vi "Tools Dialog.vi"(7 "Settings":T1, 8 "Error In":errorcluster, 10 "Context":refnum<k7>, 11 "Tools In":refnum<class "Tools.lvclass">[](array[class])) -> (0 "Error Out":errorcluster, 1 "Canceled?":bool, 2 "ID":string, 3 "Tools Out":refnum<class "Tools.lvclass">[](array[class]))   [LabVIEW 2021, in "Seq Edit Quick Drop.lvlib"]
uses:
  Seq Edit Quick Drop.lvlib
  Dependencies/Tool Menu Utility.lvlibp/Tools/Tools.lvclass
  Control Keys.ctl
  Get Modifier.vi
  <vilib>/Utility/error.llb/Trim Whitespace.vi
  <vilib>/addons/TestStand/_TSUtility.llb/TestStand - End Modal Dialog (Sequence Context).vi
  <vilib>/addons/TestStand/_TSUtility.llb/TestStand - Start Modal Dialog (Sequence Context).vi
panel:
  in  "Parameters":string
  in  "Tools":string(tree)
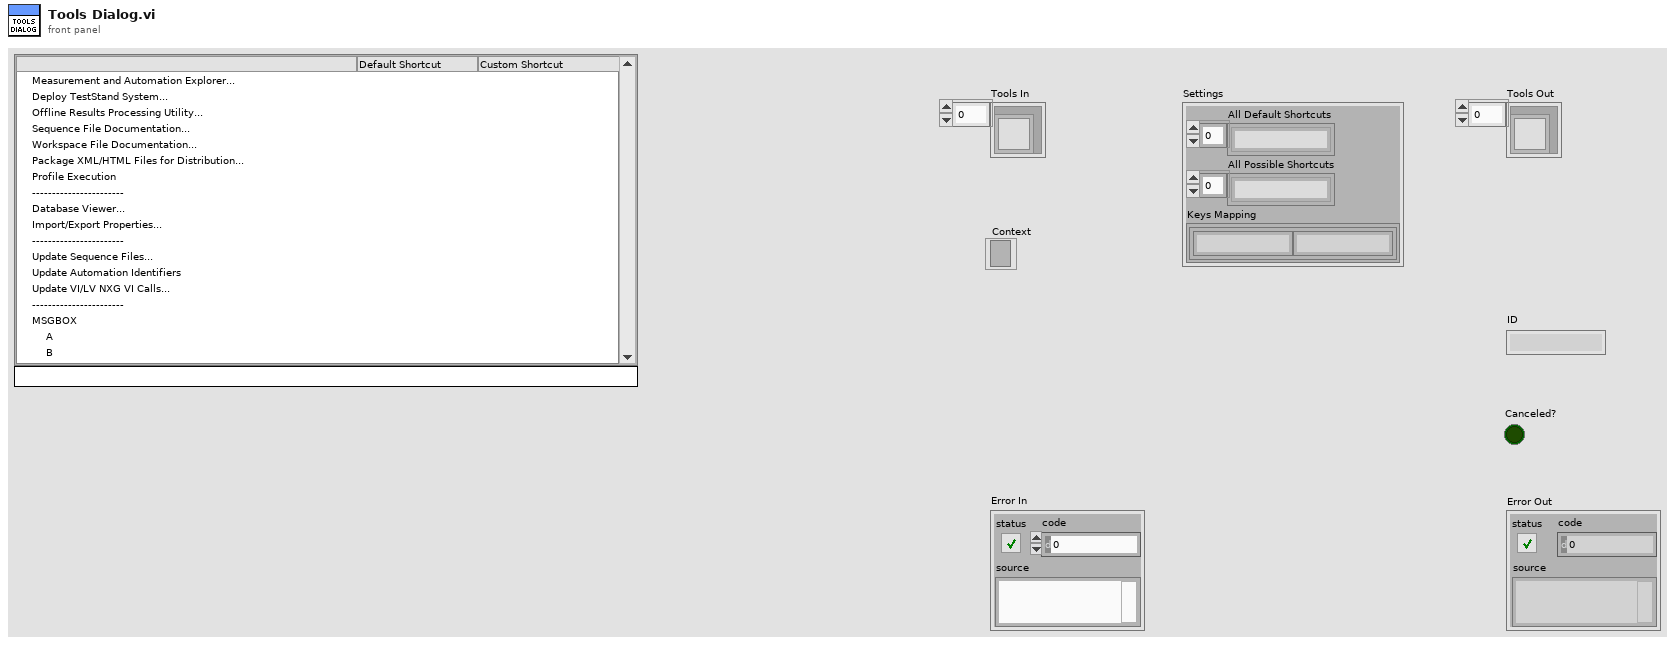
[diagram p1: front panel]
types:
  T1 = cluster{"All Default Shortcuts":string[], "All Possible Shortcuts":string[], "Keys Mapping":map{string, string}}
  T2 = typedef "Seq Edit Quick Drop.lvlib/Control Keys.ctl" = enum16{"Other", "Enter", "Escape", "Tab", "Up", "Down"}
  T3 = typedef "TestStand - Status Monitor.ctl" = cluster{"Sequence Context":refnum<k7>, "Execution":refnum<k7>, "Termination Monitor":refnum<k7>}
  T4 = cluster{"Shift":bool, "Ctrl":bool, "Alt":bool, "Cmd":bool, "Opt":bool}
  T5 = typedef "eventvkey.ctl" = enum16{"ASCII", "Enter", "Return", "Shift", "Ctrl", "Alt", "Cmd", "Opt", "Caps", "NumLock", "Clear", "Break", "Up", "Down", "Left", "Right", "Insert", "Delete", "Home", "End", "PageUp", "PageDown", "Escape", "Help", "Pause", "ScrollLock", "F1", "F2", "F3", "F4", "F5", "F6", "F7", "F8", "F9", "F10", "F11", "F12", "F13", "F14", "F15", "F16", "F17", "F18", "F19", "F20", "F21", "F22", "F23", "F24", "Play", "VolumeUp", "VolumeDown", "Mute", "Two Byte Char"}
  T6 = typedef "Seq Edit Quick Drop.lvlib/Modifiers.ctl" = enum16{"SHIFT", "CTRL", "ALT"}
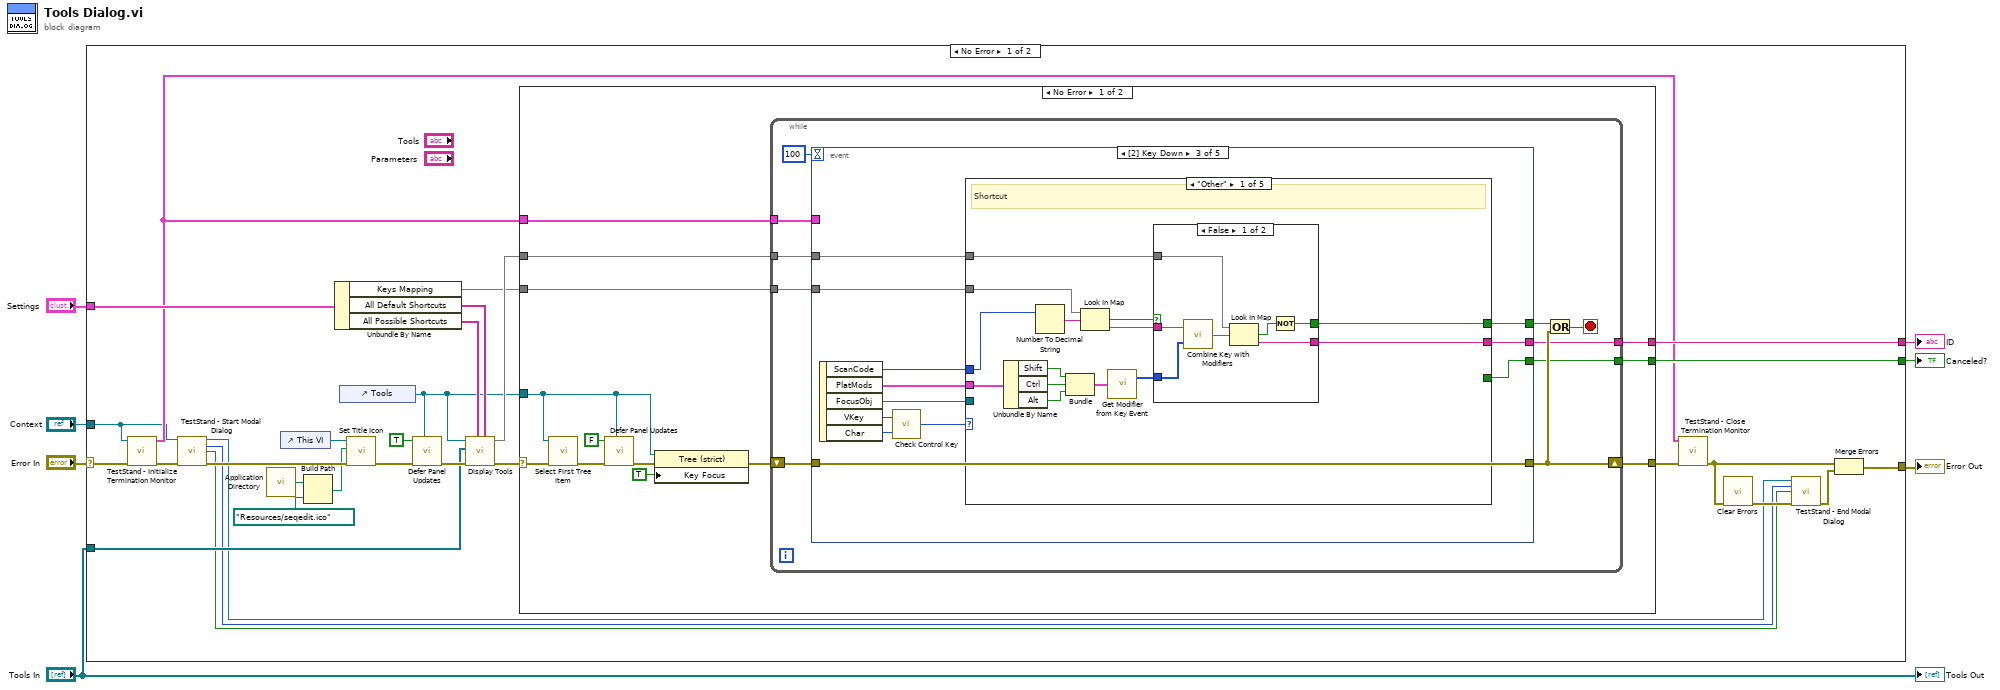
[diagram p0: block diagram]
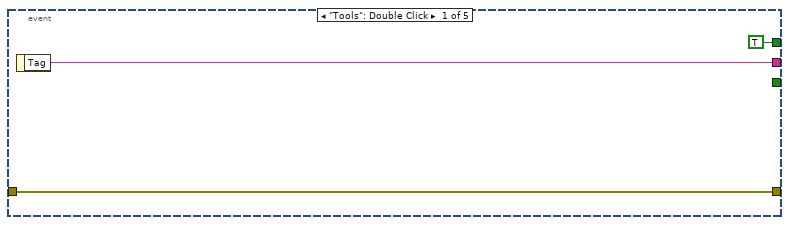
[diagram p2: hidden frame]
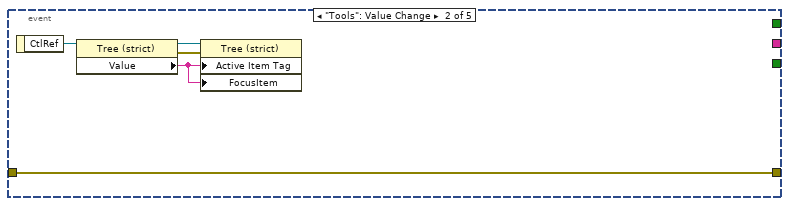
[diagram p3: hidden frame]
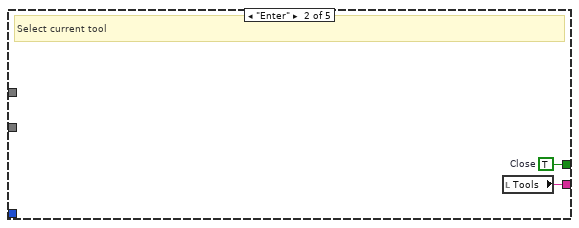
[diagram p5: hidden frame]
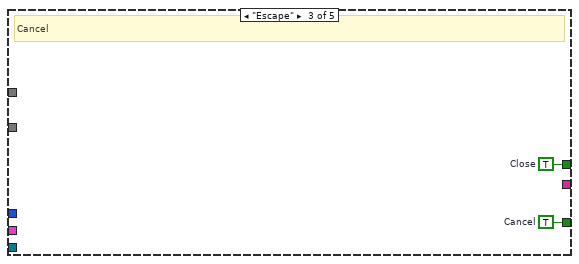
[diagram p6: hidden frame]
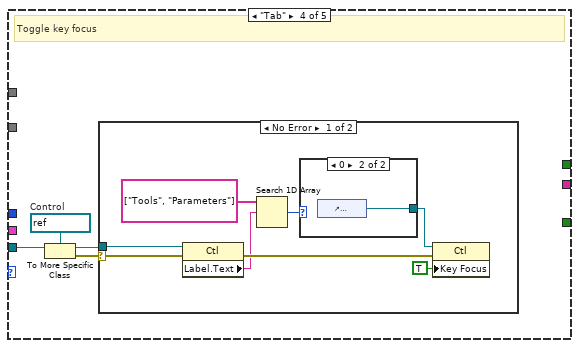
[diagram p7: hidden frame]
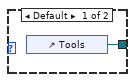
[diagram p8: hidden frame]
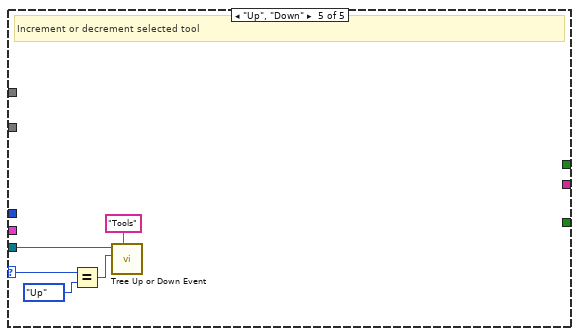
[diagram p10: hidden frame]
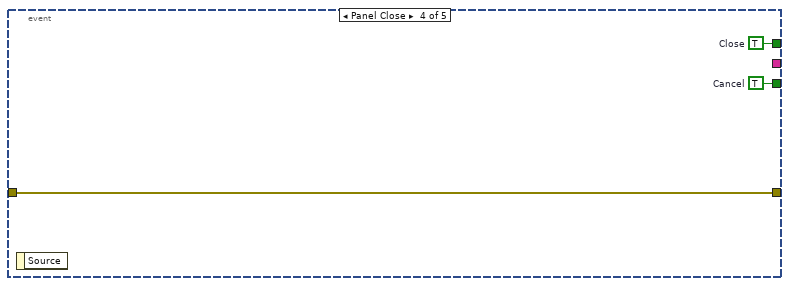
[diagram p11: hidden frame]
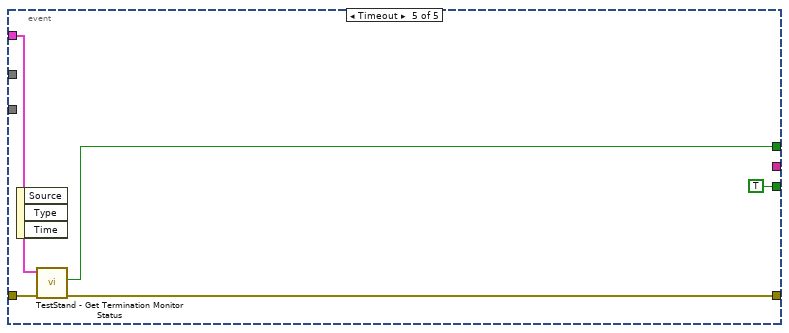
[diagram p12: hidden frame]
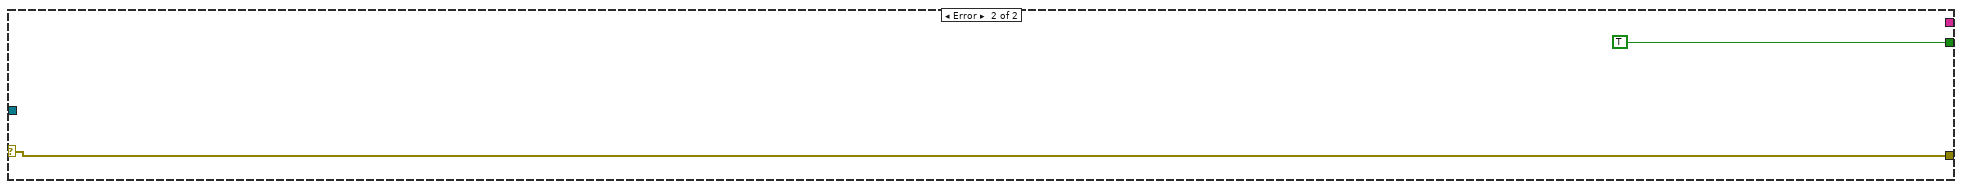
[diagram p14: hidden frame]
diagram:
  n1 = case shown="No Error" "Error In" {
    selector: "Error In" -> [w8 w135]
    tunnel: [w32 _] -> w7
    tunnel: "Tools In" -> [w31 _]
    tunnel: "Settings" -> [w30 _]
    tunnel: [w26 TRUE ("Cancel")] -> w4
    tunnel: [w24 w135] -> w3
    tunnel: "Context" -> [w14 _]
    frame No Error {
      n2 = call <vilib>:"TestStand - Initialize Termination Monitor.vi"("error in (no error)"=w8, "Sequence Context In"=w14) -> ("error out"=w21:errorcluster, "Status Monitor Out"=w19:T3)  [unwired: 8 in]
      n3 = call-poly <vilib>:"TestStand - Start Modal Dialog.vi"("Sequence Context In"=w14, "error in (no error)"=w21) -> ("Sequence Context Out"=w18:refnum<k7>, "Modal ID"=w23:i32, "VI Originally Open"=w22:bool, "error out"=w37:errorcluster)  [unwired: 9 in, 1 out]
      n4 = call <vilib>:"Application Directory.vi"() -> ("Application Directory"=w12:path)
      n5 = control-ref of="This VI"() -> (w13:refnum<vi>)
      n6 = Build Path(base path=w12, name or relative path=path "Resources/seqedit.ico") -> (appended path=w10:path)
      n7 = Unbundle By Name(w30) -> ("Keys Mapping"=w27:map{string, string}, "All Default Shortcuts"=w28:string[], "All Possible Shortcuts"=w29:string[])
      n8 = control-ref of="Tools"() -> (w15:refnum<vi>)
      n9 = call "Set Title Icon.vi"("Error In"=w37, "Icon Path"=w10, "VI Reference"=w13) -> ("Error Out"=w9:errorcluster)  [unwired: 8 in]
      n10 = call "Defer Panel Updates.vi"("Control"=w15, "Error In"=w9, "Defer Panel Updates"=TRUE) -> ("Error Out"=w34:errorcluster)  [unwired: 8 in]
      n11 = call "Display Tools.vi"("All Default Shortcuts"=w28, "All Possible Shortcuts"=w29, "Error In"=w34, "Tools"=w31, "Tools Tree Control"=w15) -> ("Error Out"=w35:errorcluster, "Shortcuts"=w33:map{string, string})  [unwired: 5 in]
      n12 = case shown="No Error" w35 {
        selector: w35 -> [w47 w133]
        tunnel: w33 -> [w49 _]
        tunnel: w15 -> [w41 _]
        tunnel: [w46 _] -> w32
        tunnel: w27 -> [w48 _]
        tunnel: [w45 _] -> w26
        tunnel: w19 -> [w39 _]
        tunnel: [w38 w133] -> w20
        frame No Error {
          n13 = call "Select First Tree Item.vi"("error in (no error)"=w47, "TreeControl in"=w41) -> ("error out"=w50:errorcluster)  [unwired: 8 in, 1 out]
          n14 = call "Defer Panel Updates.vi"("Control"=w41, "Error In"=w50, "Defer Panel Updates"=FALSE) -> ("Error Out"=w44:errorcluster)  [unwired: 8 in]
          n15 = property class="Tree (strict)"(reference=w41, error in=w44, "Key Focus"=TRUE) -> (error out=w42:errorcluster)  [unwired: 1 out]
          n16 = while {
            tunnel: [w59] -> w45
            tunnel: [w58] -> w46
            tunnel: w48 -> [w57]
            tunnel: w49 -> [w56]
            tunnel: w39 -> [w55]
            shift-right: [w60] -> w38
            shift-left: w42 -> [w53]
            stop <- w51 stop-if-true
            n17 = event shown="[2] Key Down" {
              selector: _ -> [_ _ _ _ _]
              dyn-events: _ -> [_ _ _ _ _]
              timeout: 100 -> [_ _ _ _ _]
              tunnel: [_ _ w75 w127 TRUE ("Cancel")] -> w59
              tunnel: [w63 _ w76 _ _] -> w58
              tunnel: w57 -> [_ _ w79 _ _]
              tunnel: [TRUE ("Close") _ w74 w126 w132] -> w52
              tunnel: w56 -> [_ _ w73 _ _]
              tunnel: w55 -> [_ _ _ _ w130]
              tunnel: w53 -> [w61 w64 w69 w125 w129]
              tunnel: [w61 w64 w69 w125 w128] -> w60
              event "Tools": Double Click {
                n18 = event-data() -> ("Tag"=w63:string)  [unwired: 1 in]
              }
              event "Tools": Value Change {
                n19 = event-data() -> ("CtlRef"=w68:refnum<vi>)  [unwired: 1 in]
                n20 = property class="Tree (strict)"(reference=w68) -> (reference out=w67:refnum<vi>, error out=w66:errorcluster, "Value"=w65:string)  [unwired: 1 in]
                n21 = property class="Tree (strict)"(reference=w67, error in=w66, "Active Item Tag"=w65, "FocusItem"=w65) -> ()  [unwired: 2 out]
              }
              event Key Down {
                n22 = event-data() -> ("ScanCode"=w80:i16, "PlatMods"=w78:T4, "FocusObj"=w70:refnum<vi>, "VKey"=w71:T5, "Char"=w72:i16)  [unwired: 1 in]
                n23 = call "Check Control Key.vi"("Char"=w72, "VKey"=w71) -> ("Control Key"=w77:T2)
                n24 = case shown="\"Other\"" w77 {
                  selector: w77 -> [_ _ _ _ w122]
                  tunnel: w80 -> [w94 _ _ _ _]
                  tunnel: w79 -> [w92 _ _ _ _]
                  tunnel: w78 -> [w88 _ _ _ _]
                  tunnel: [w82 w103 _ _ _] -> w76
                  tunnel: [_ _ w105 _ _] -> w75
                  tunnel: [w81 w102 w104 _ _] -> w74
                  tunnel: w70 -> [_ _ _ w109 w124]
                  tunnel: w73 -> [w83 _ _ _ _]
                  frame "Other" {
                    # "Shortcut"
                    n25 = Unbundle By Name(w88) -> ("Shift"=w87:bool, "Ctrl"=w86:bool, "Alt"=w85:bool)
                    n26 = Number To Decimal String(number=w94) -> (decimal integer string=w93:string)  [unwired: 1 in]
                    n27 = Bundle("Shift"=w87, "Ctrl"=w86, "Alt"=w85) -> (w84:cluster{"Shift":bool, "Ctrl":bool, "Alt":bool})  [unwired: 1 in]
                    n28 = Look In Map(map=w92, key=w93) -> (key not found?=w91:bool, value=w89:string)  [unwired: 1 in]
                    n29 = call "Get Modifier from Key Event.vi"("Modifiers"=w84) -> ("Modifiers"=w90:T6[])  [unwired: 1 out]
                    n30 = case shown="False" w91 {
                      tunnel: w90 -> [w101 _]
                      tunnel: w89 -> [w100 _]
                      tunnel: w83 -> [w98 _]
                      tunnel: [w97 _] -> w82
                      tunnel: [w95 _] -> w81
                      frame False {
                        n31 = call "Combine Key with Modifiers.vi"("Modifiers"=w101, "Key"=w100) -> ("Combined"=w99:string)
                        n32 = Look In Map(map=w98, key=w99) -> (key not found?=w96:bool, value=w97:string)  [unwired: 1 in]
                        n33 = Not(x=w96) -> (.not. x?=w95:bool)
                      }
                      frame True {
                      }
                    }
                  }
                  frame "Enter" {
                    w102 = TRUE  # Close
                    # "Select current tool"
                    n34 = local read "Tools"() -> (w103:string)
                  }
                  frame "Escape" {
                    w104 = TRUE  # Close
                    w105 = TRUE  # Cancel
                    # "Cancel"
                  }
                  frame "Tab" {
                    w108 = refnum<vi> refnum  # Control
                    # "Toggle key focus"
                    n35 = To More Specific Class(target class=w108, reference=w109) -> (specific class reference=w106:refnum<vi>, error out=w107:errorcluster)  [unwired: 1 in]
                    n36 = case shown="No Error" w107 {
                      selector: w107 -> [w115 _]
                      tunnel: w106 -> [w116 _]
                      frame No Error {
                        n37 = property class="Ctl"(reference=w116, error in=w115) -> (error out=w117:errorcluster, "Label.Text"=w114:string)  [unwired: 1 out]
                        n38 = Search 1D Array(1D array=string[] ["Tools", "Parameters"], element=w114) -> (index of element=w112:i32)  [unwired: 1 in]
                        n39 = case shown="0" w112 {
                          tunnel: [w118 w119] -> w111
                          frame Default {
                            n40 = control-ref of="Tools"() -> (w118:refnum<vi>)
                          }
                          frame 0 {
                            n41 = control-ref of="Parameters"() -> (w119:refnum<vi>)
                          }
                        }
                        n42 = property class="Ctl"(reference=w111, error in=w117, "Key Focus"=TRUE) -> ()  [unwired: 2 out]
                      }
                      frame Error {
                      }
                    }
                  }
                  frame "Up", "Down" {
                    # "Increment or decrement selected tool"
                    n43 = Equal?(x=w122, y=Control_Keys."Up") -> (x = y?=w120:bool)
                    n44 = call "Tree Up or Down Event.vi"("Label"="Tools", "Up?"=w120, "GObject"=w124) -> ()  [unwired: 9 in]
                  }
                }
              }
              event Panel Close {
                w126 = TRUE  # Close
                w127 = TRUE  # Cancel
                n45 = event-data() -> ()  [unwired: 1 in, 1 out]
              }
              event Timeout {
                n46 = event-data() -> ()  [unwired: 1 in, 3 out]
                n47 = call <vilib>:"TestStand - Get Termination Monitor Status.vi"("error in (no error)"=w129, "Status Monitor In"=w130) -> ("error out"=w128:errorcluster, "Terminating or Aborting"=w132:bool)  [unwired: 7 in, 1 out]
              }
            }
            n48 = Or(x=w52, y=w60) -> (x .or. y?=w51:bool)
          }
        }
        frame Error {
        }
      }
      n49 = call <vilib>:"TestStand - Close Termination Monitor.vi"("error in (no error)"=w20, "Status Monitor In"=w19) -> ("error out"=w17:errorcluster)  [unwired: 9 in]
      n50 = call <vilib>:"Clear Errors.vi"("error in (no error)"=w17) -> ("error out"=w36:errorcluster)  [unwired: 5 in, 1 out]
      n51 = call-poly <vilib>:"TestStand - End Modal Dialog.vi"("Sequence Context In"=w18, "Modal ID"=w23, "VI Originally Open"=w22, "error in (no error)"=w36) -> ("error out"=w16:errorcluster)  [unwired: 11 in]
      n52 = Merge Errors(w17, w16) -> (w24:errorcluster)
    }
    frame Error {
    }
  }
  "Error Out" <- w3
  "Canceled?" <- w4
  "ID" <- w7
  "Tools Out" <- "Tools In"
